vi "Generate Sound.vi"() -> ()   [LabVIEW 2022 SP3]
doc: "This VI illustrates how to generate and play sine, square, sawtooth and triangle waveforms. You can change the frequency and type of the waveform generated as it plays continuously."
uses:
  WhiteNoise.ctl
  <vilib>/sound2/lvsound2.llb/Sampling Mode.ctl
  <vilib>/sound2/lvsound2.llb/Sound Data Format.ctl
  <vilib>/DAQmx/write.llb/DAQmx Write (Analog 1D DBL 1Chan NSamp).vi
  <vilib>/DAQmx/create/channels.llb/DAQmx Create Channel (AO-Voltage-Basic).vi
  <vilib>/DAQmx/configure/timing.llb/DAQmx Timing (Sample Clock).vi
  <vilib>/sound2/lvsound2.llb/Sound Output Set Volume (Single).vi
  <vilib>/sound2/lvsound2.llb/Sound Output Write (DBL).vi
  <vilib>/DAQmx/miscellaneous.llb/DAQmx Fill In Error Info.vi
  <resource>/objmgr/daqmx.rc
  <vilib>/measure/NI_MABase.lvlib
panel:
  in  "Tab Control":enum32{"White Noise", "Harmonic"}(tab)
  in  "Cluster":T2={"Seed"=0.0, "Standard Deviation"=0.275, "Reset"=FALSE, "Iterator"=1.0, "Seed"=-1, "Stop 4"=FALSE} {"Standard Deviation" min=0.001 max=0.3 format="%0.2p"}
  in  "Stop 4":bool
  in  "Output Array":T3(array[cluster])=[{"Waveform Type"=0, "Amplitude"=1.0, "Frequency"=10.0}] {"Frequency" format="%0.2p"; "Amplitude" format="%0.2p"; "Waveform Type" items=["Sine Wave", "Triangle Wave", "Square Wave", "Sawtooth Wave"]}
  out "Active Control":waveform(dbl)[](graph)
  in  "Setpoint":dbl
  in  "Gain":dbl min=0.0 step=0.01
  out "number of samples written per channel":u32
  in  "Active Control":bool
  in  "Volume":dbl(slide)=50.0 scale=0.0..100.0
  out "Generated Sound":waveform(dbl)[](graph)
  in  "Device ID":u32
  # "Runtime"
  # "Filter"
  # "Waveform Settings"
  # "The number of elements in the waveform array must equal the number of channels in the task."
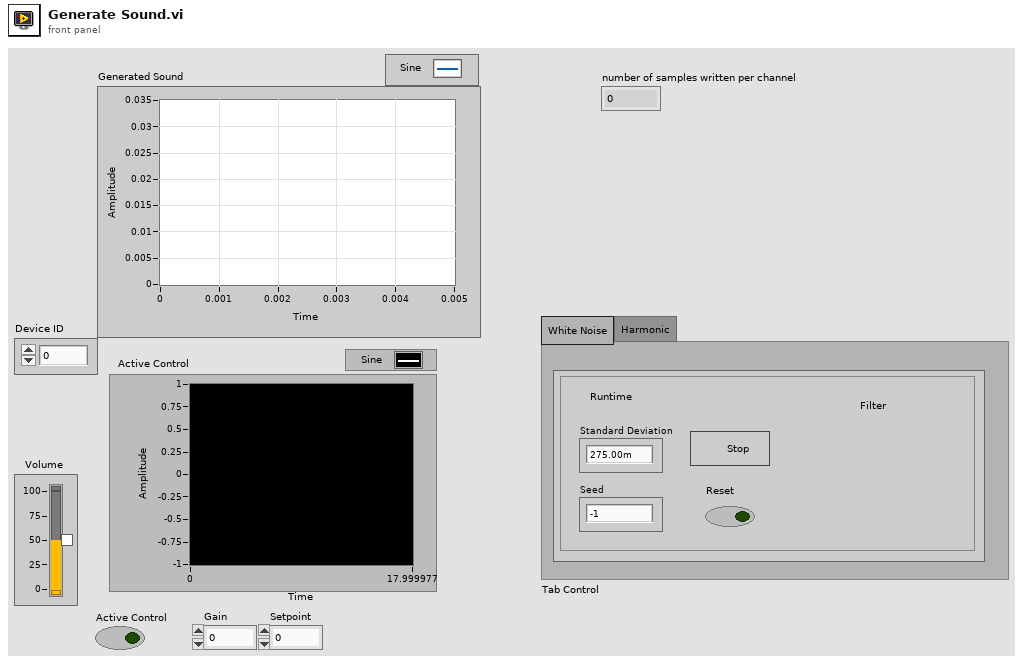
[diagram p1: front panel]
types:
  T1 = typedef "WhiteNoise.ctl" = dbl
  T2 = cluster{"Seed":T1, "Standard Deviation":dbl, "Reset":bool, "Iterator":dbl, "Seed":i8, "Stop 4":bool}
  T3 = cluster{"Waveform Type":u16, "Amplitude":dbl, "Frequency":dbl}[]
  T4 = typedef "Sound Data Format.ctl" = cluster{"sample rate (S/s)":dbl, "number of channels":i32, "bits per sample":i32}
  T5 = typedef "Sampling Mode.ctl" = i32
  T6 = typedef "Sound Output Task ID.ctl" = u32
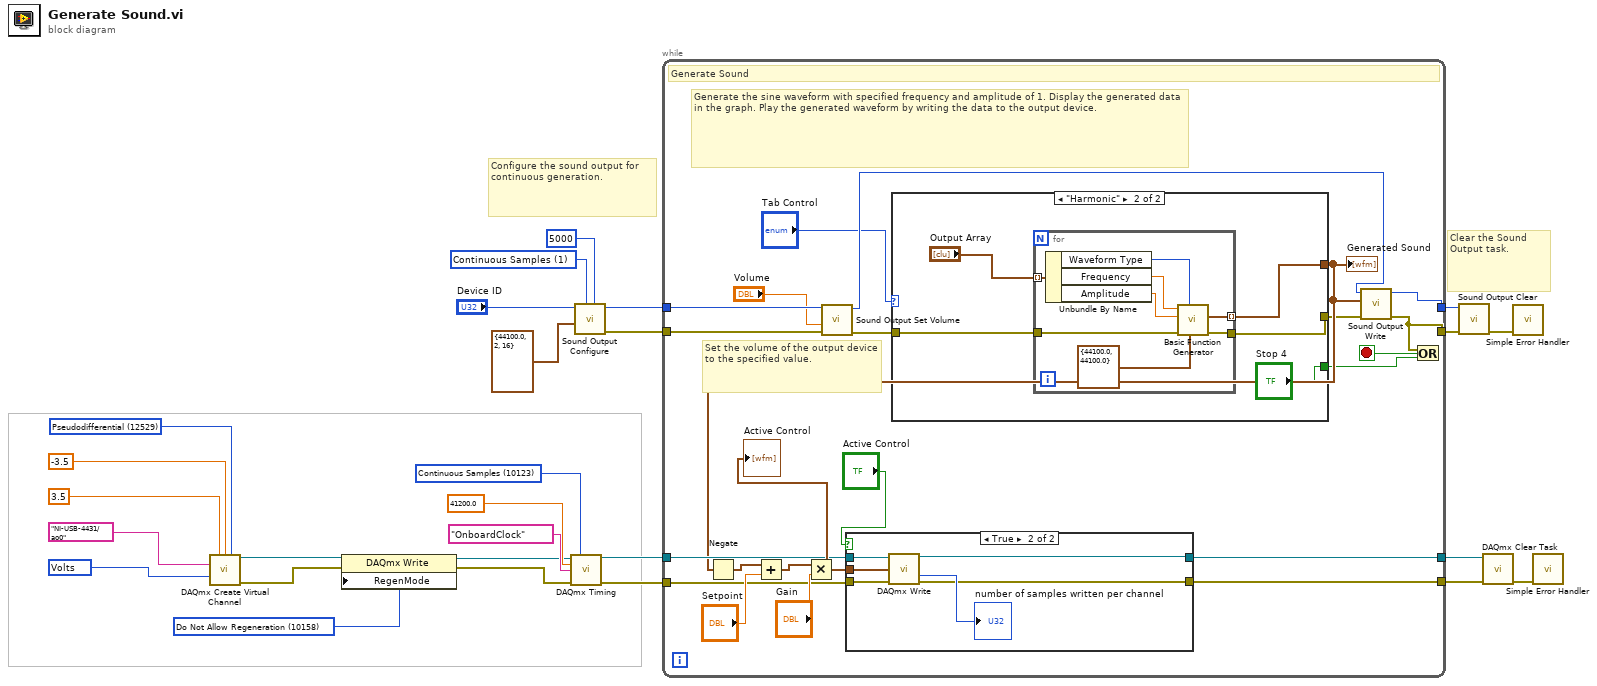
[diagram p0: block diagram]
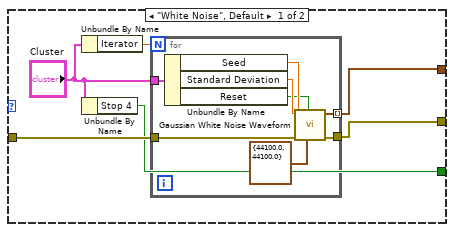
[diagram p2: hidden frame]
diagram:
  w6 = 10123 items=["Finite Samples"=10178, "Continuous Samples"=10123, "Hardware Timed Single Point"=12522] ("sample mode")
  w10 = 10158 items=["Allow Regeneration"=10097, "Do Not Allow Regeneration"=10158] ("RegenMode")
  w16 = 12529 items=["Default"=-1, "RSE"=10083, "Differential"=10106, "Pseudodifferential"=12529] ("output terminal configuration")
  w14 = 10348 items=["Volts"=10348, "From Custom Scale"=10065] ("units")
  w22 = T5 1 items=["Finite Samples", "Continuous Samples"] ("sample mode")
  # "Configure the sound output for continuous generation."
  # "Clear the Sound Output task."
  n1 = call-poly <vilib>:"DAQmx Create Virtual Channel.vi"("maximum value"=3.5, "minimum value"=-3.5, "output terminal configuration"=w16, "physical channels"=tag "NI-USB-4431/ao0", "units"=w14) -> ("task out"=w9:refnum<k21>, "error out"=w11:errorcluster)  [unwired: 9 in]
  n2 = property class="DAQmx Write"(reference=w9, error in=w11, "RegenMode"=w10) -> (reference out=w7:refnum<k21>, error out=w8:errorcluster)
  n3 = call-poly <vilib>:"DAQmx Timing.vi"("task/channels in"=w7, "sample mode"=w6, "rate"=41200.0 ("Sample Rate"), "source"=tag "OnboardClock" ("Sample Clock Source"), "error in"=w8) -> ("task out"=w5:refnum<k21>, "error out"=w4:errorcluster)  [unwired: 9 in]
  n4 = call <vilib>:"Sound Output Configure.vi"("number of samples/ch"=5000 ("Number of Samples/ch"), "sample mode"=w22, "sound format"=T4 {"sample rate (S/s)"=44100.0, "number of channels"=2, "bits per sample"=16} ("Sound Format"), "device ID"="Device ID") -> ("error out"=w27:errorcluster, "task ID"=w26:T6)  [unwired: 6 in]
  n5 = while {
    tunnel: w26 -> [w46]
    tunnel: [w49] -> w24
    tunnel: w27 -> [w47]
    tunnel: [w44] -> w25
    tunnel: w5 -> [w37]
    tunnel: w4 -> [w36]
    tunnel: [w34] -> w2
    tunnel: [w33] -> w1
    stop <- w48 stop-if-true
    # "Set the volume of the output device to the specified value."
    # "Generate the sine waveform with specified frequency and amplitude of 1. Display the generated data in the graph. Play the generated waveform by writing the data to the output device."
    # "Generate Sound"
    n6 = call-poly <vilib>:"Sound Output Set Volume.vi"("error in (no error)"=w47, "volume"="Volume", "task ID"=w46) -> ("error out"=w31:errorcluster, "task ID out"=w29:T6)  [unwired: 7 in]
    n7 = case shown="\"Harmonic\"" "Tab Control" {
      tunnel: [w50 w65] -> w35
      tunnel: [w53 w66] -> w32
      tunnel: w31 -> [w52 w67]
      tunnel: [w51 "Stop 4"] -> w30
      frame "White Noise", Default {
        n8 = Unbundle By Name("Cluster") -> ("Iterator"=w54:dbl)
        n9 = Unbundle By Name("Cluster") -> ("Stop 4"=w51:bool)
        n10 = for {
          N: w54 -> [_]
          tunnel: w52 -> [w63]
          tunnel: [w62] -> w53
          tunnel: "Cluster" -> [w61]
          tunnel: [w60] -> w50 mode=indexing
          n11 = Unbundle By Name(w61) -> ("Seed"=w59:T1, "Standard Deviation"=w58:dbl, "Reset"=w57:bool)
          n12 = call <vilib>:"Gaussian White Noise Waveform.vi"("sampling info"=cluster{"Fs":dbl, "#s":dbl} {"Fs"=44100.0, "#s"=44100.0}, "reset signal"=w57, "error in (no error)"=w63, "seed"=w59, "standard deviation"=w58) -> ("error out"=w62:errorcluster, "signal out"=w60:waveform(dbl))  [unwired: 5 in]
        }
      }
      frame "Harmonic" {
        n13 = for {
          tunnel: w67 -> [w76]
          tunnel: [w75] -> w66
          tunnel: "Output Array" -> [w74] mode=indexing
          tunnel: [w70] -> w65 mode=indexing
          n14 = Unbundle By Name(w74) -> ("Waveform Type"=w73:u16, "Frequency"=w72:dbl, "Amplitude"=w71:dbl)
          n15 = call <vilib>:"Basic Function Generator.vi"("sampling info"=cluster{"Fs":dbl, "#s":dbl} {"Fs"=44100.0, "#s"=44100.0}, "signal type"=w73, "error in (no error)"=w76, "amplitude"=w71, "frequency"=w72) -> ("error out"=w75:errorcluster, "signal out"=w70:waveform(dbl))  [unwired: 4 in, 1 out]
        }
      }
    }
    "Generated Sound" <- w35
    n16 = Negate(x=w35) -> (-x=w41:waveform(dbl)[])
    n17 = Add(x=w41, y="Setpoint") -> (x+y=w42:waveform(dbl)[])
    n18 = Multiply(x=w42, y="Gain") -> (x*y=w38:waveform(dbl)[])
    "Active Control" <- w38
    n19 = case shown="True" "Active Control" {
      tunnel: w36 -> [w78 w82]
      tunnel: [w77 w79] -> w33
      tunnel: [w78 w80] -> w34
      tunnel: w37 -> [w77 w84]
      tunnel: w38 -> [_ w83]
      frame False {
      }
      frame True {
        n20 = call-poly <vilib>:"DAQmx Write.vi"("task/channels in"=w84, "data"=w83, "error in"=w82) -> ("task out"=w79:refnum<k21>, "number of samples written per channel"=→"number of samples written per channel":u32, "error out"=w80:errorcluster)  [unwired: 10 in]
      }
    }
    n21 = call-poly <vilib>:"Sound Output Write.vi"("error in (no error)"=w32, "data"=w35, "task ID"=w29) -> ("error out"=w44:errorcluster, "task ID out"=w49:T6)  [unwired: 7 in]
    n22 = Or(x=w44, y=w30) -> (x .or. y?=w48:bool)
  }
  n23 = call <vilib>:"Sound Output Clear.vi"("error in (no error)"=w25, "task ID"=w24) -> ("error out"=w20:errorcluster)  [unwired: 9 in]
  n24 = call <vilib>:"DAQmx Clear Task.vi"("task in"=w1, "error in"=w2) -> ("error out"=w3:errorcluster)  [unwired: 13 in]
  n25 = call <vilib>:"Simple Error Handler.vi"("error in (no error)"=w20) -> ()  [unwired: 4 in, 5 out]
  n26 = call <vilib>:"Simple Error Handler.vi"("error in (no error)"=w3) -> ()  [unwired: 4 in, 5 out]
